vi "F Dwf Analog Out Node Offset Info.vi"(6 "pMax":dbl, 7 "pMin":dbl, 8 "error in (no error)":errorcluster, 9 "node":i32, 10 "idxChannel":i32, 11 "hdwf":i32) -> (0 "error out":errorcluster, 3 "function return":i32, 4 "pMax out":dbl, 5 "pMin out":dbl)   [LabVIEW 2021, in "Olasdwf.lvlib"]
doc: "DWFAPI int FDwfAnalogOutNodeOffsetInfo(HDWF hdwf, int idxChannel, AnalogOutNode node, double *pMin, double *pMax);"
uses:
  Olasdwf.lvlib
  Windows/System32/dwf.dll
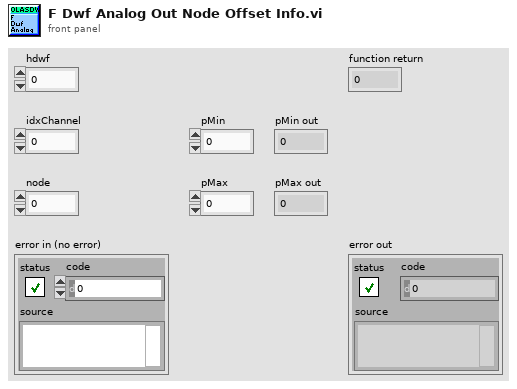
[diagram p1: front panel]
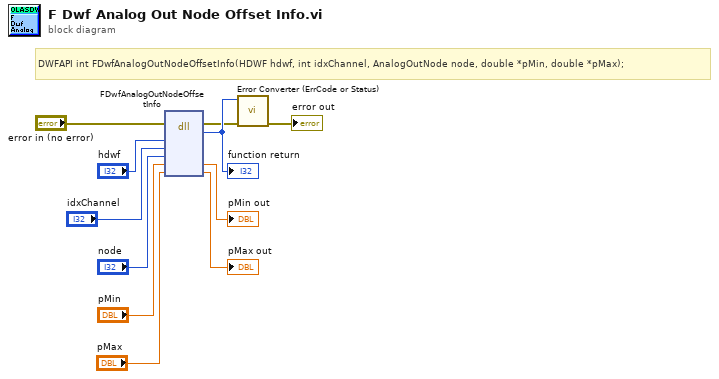
[diagram p0: block diagram]
diagram:
  # "DWFAPI int FDwfAnalogOutNodeOffsetInfo(HDWF hdwf, int idxChannel, AnalogOutNode node, double *pMin, double *pMax);"
  n1 = dll-call lib="/Windows/System32/dwf.*" fn="FDwfAnalogOutNodeOffsetInfo"(error in="error in (no error)", "hdwf"="hdwf", "idxChannel"="idxChannel", "node"="node", "pMin"="pMin", "pMax"="pMax") -> (error out=w2:errorcluster, w11:i32, "pMin"=→"pMin out":dbl, "pMax"=→"pMax out":dbl)  [unwired: 5 in, 1 out]
  "function return" <- w11
  n2 = call "Error Converter (ErrCode or Status).vi"("error in (no error)"=w2, "error code"=w11) -> ("error out"=→"error out":errorcluster)  [unwired: 9 in]
